vi "Thruster8.vi"(0 "period":dbl=10.0, 1 "Thruster 2":bool, 3 "Truster1":bool, 4 "Floating":bool, 5 "Thruster 3":bool, 6 "Thruster 8":bool, 7 "task in":refnum<k21>, 9 "Thruster 4":bool, 10 "Thruster 7":bool, 11 "Duty Cycle":dbl=0.5, 12 "Thruster 5":bool, 13 "error in":errorcluster, 14 "Thruster 6":bool) -> (8 "task out":refnum<k21>, 15 "error out":errorcluster)   [LabVIEW 2012]
doc: "I. Description:\nThis example demonstrates how to write values to a digital output channel.\n\nII. Instructions for Running:\n1. Select the digital lines on the DAQ device to be written.\n2. Select a value to write.\nNote: The array control is sized for 8 lines, if using a different amount of lines, change the number of elements in the array to equal the number of lines chosen.\n\nIII. Block Diagram Steps:\n1. Create a Digital Output channel. Use one channel for all lines. You can alternatively use one channel for each line, but then use a different polymorphic version of the DAQmx Write VI.\n2. Call the Start VI to start the task.\n3. Write the digital Boolean array data in a loop until the user hits the stop button or an error occurs. This write VI writes a single sample of digital data on demand, so no timeout is necessary.\n4. Call the Clear Task VI to clear the Task.\n5. Use the popup dialog box to display an error or warning if any.\n\nIV. I/O Connections Overview:\nMake sure your signal output terminals match the Lines I/O Control. In this case wire the item to receive the signal to the first eight digital lines on your DAQ Device."
uses:
  <vilib>/DAQmx/write.llb/DAQmx Write (Digital 1D Bool 1Chan 1Samp).vi
  <vilib>/DAQmx/miscellaneous.llb/DAQmx Fill In Error Info.vi
panel:
  # "Thruster and Air-Floating Control"
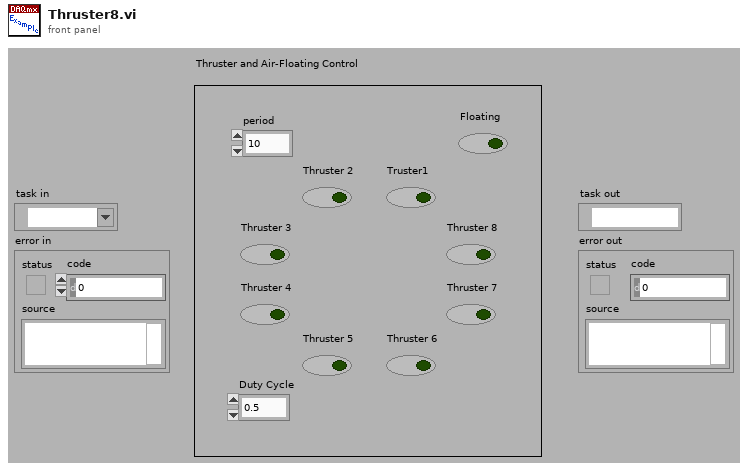
[diagram p1: front panel]
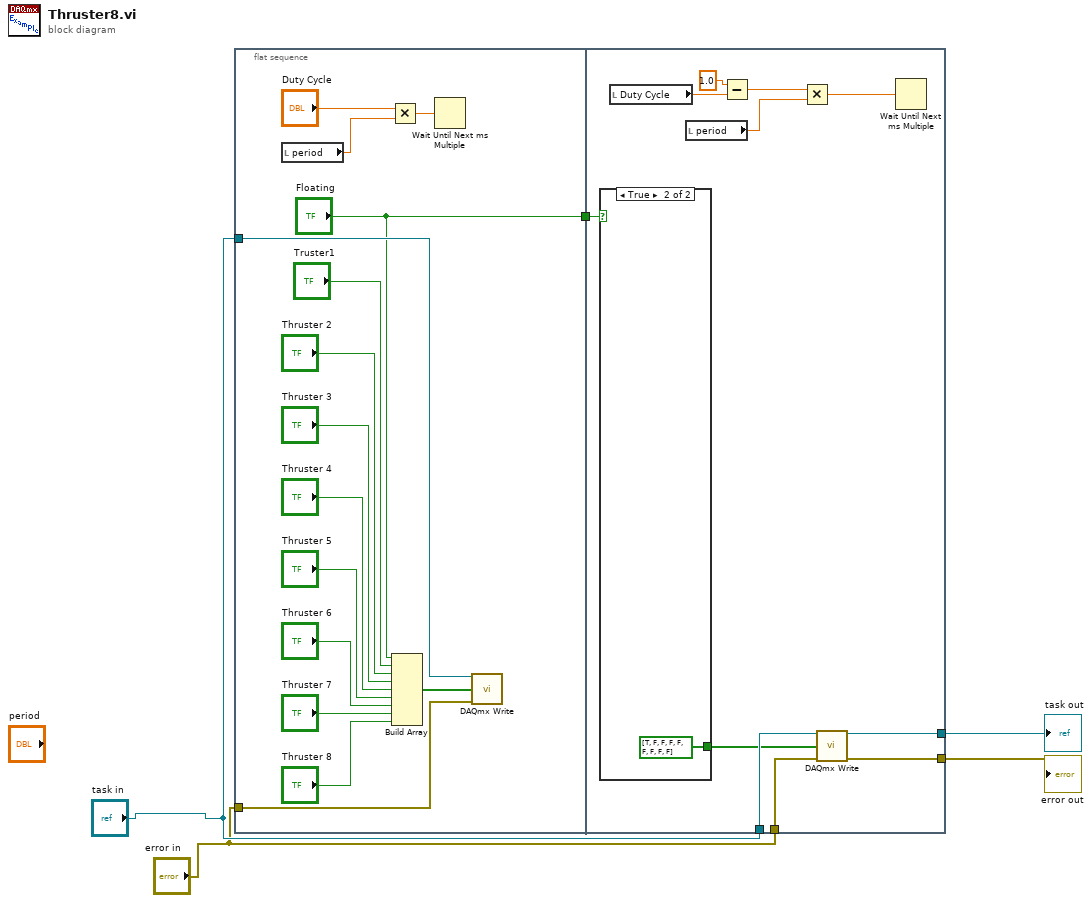
[diagram p0: block diagram]
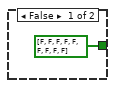
[diagram p2: hidden frame]
diagram:
  n1 = flat-sequence {
    tunnel: "task in" -> [w20]
    tunnel: "error in" -> [w19]
    tunnel: ["Floating"] -> w3
    tunnel: "task in" -> [w31]
    tunnel: "error in" -> [w30]
    tunnel: [w29] -> w5
    tunnel: [w28] -> w4
    tunnel: w3 -> [w22]
    frame #0 {
      n2 = local read "period"() -> (w17:dbl)
      n3 = Multiply(x="Duty Cycle", y=w17) -> (x*y=w16:dbl)
      n4 = Build Array("Floating", "Truster1", "Thruster 2", "Thruster 3", "Thruster 4", "Thruster 5", "Thruster 6", "Thruster 7", "Thruster 8") -> (w7:bool[])
      n5 = Wait Until Next ms Multiple(millisecond multiple=w16) -> ()  [unwired: 1 out]
      n6 = call-poly <vilib>:"DAQmx Write.vi"("task/channels in"=w20, "data"=w7, "error in"=w19) -> ()  [unwired: 10 in, 3 out]
    }
    frame #1 {
      n7 = case shown="True" w22 {
        tunnel: [bool[] [FALSE, FALSE, FALSE, FALSE, FALSE, FALSE, FALSE, FALSE, FALSE] ("Data to Write 2") bool[] [TRUE, FALSE, FALSE, FALSE, FALSE, FALSE, FALSE, FALSE, FALSE] ("Data to Write 2")] -> w21
        frame False {
        }
        frame True {
        }
      }
      n8 = local read "Duty Cycle"() -> (w23:dbl)
      n9 = local read "period"() -> (w25:dbl)
      n10 = Subtract(x=1.0, y=w23) -> (x-y=w26:dbl)
      n11 = Multiply(x=w26, y=w25) -> (x*y=w24:dbl)
      n12 = call-poly <vilib>:"DAQmx Write.vi"("task/channels in"=w31, "data"=w21, "error in"=w30) -> ("task out"=w29:refnum<k21>, "error out"=w28:errorcluster)  [unwired: 10 in, 1 out]
      n13 = Wait Until Next ms Multiple(millisecond multiple=w24) -> ()  [unwired: 1 out]
    }
  }
  "task out" <- w5
  "error out" <- w4
